vi "Timer Updated.vi"(8 "error in (no error)":errorcluster, 10 "Timer":timestamp format="%^<%H:%M:%S%3u>T", 11 "Module ID":i32=-1) -> (0 "error out":errorcluster)   [LabVIEW 2018, in "Timer Module.lvlib"]
doc: "Timer module broadcasts every time the timer increments its value.\n_____\nCreated using Delacor QMH Event Scripter 4.1.0.76."
uses:
  Timer Module.lvlib
  Timer Updated Argument--cluster.ctl
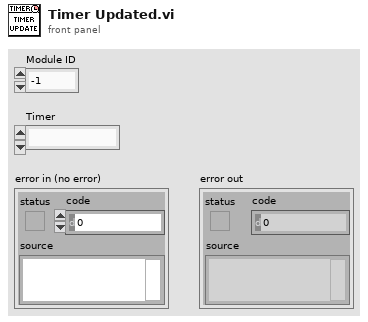
[diagram p1: front panel]
types:
  T1 = typedef "Timer Module.lvlib/Timer Updated Argument--cluster.ctl" = cluster{"Module ID":i32, "Timer":timestamp}
  T2 = typedef "Timer Module.lvlib/Broadcast Events--cluster.ctl" = cluster{"Module Did Init":refnum<user-event>, "Status Updated":refnum<user-event>, "Error Reported":refnum<user-event>, "Module Did Stop":refnum<user-event>, "Update Module Execution Status":refnum<user-event>, "Timer Updated":refnum<user-event>}
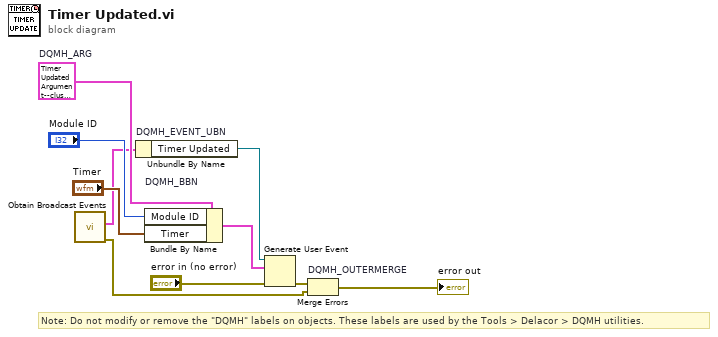
[diagram p0: block diagram]
diagram:
  w5 = T1 {"Module ID"=-1, "Timer"=timestamp(0 s since 1904-01-01)}  # DQMH_ARG
  # "Note: Do not modify or remove the \"DQMH\" labels on objects. These labels are used by the Tools > Delacor > DQMH utilities."
  n1 = call "Obtain Broadcast Events.vi"() -> ("error out"=w2:errorcluster, "Timer Module Broadcast Events"=w1:T2)  [unwired: 10 in]
  n2 = Unbundle By Name "DQMH_EVENT_UBN"(w1) -> ("Timer Updated"=w7:refnum<user-event>)
  n3 = Bundle By Name "DQMH_BBN"(cluster=w5, "Module ID"="Module ID", "Timer"="Timer") -> (w8:T1)
  n4 = Generate User Event(user event=w7, event data cluster=w8, error in="error in (no error)") -> (error out=w6:errorcluster)  [unwired: 1 in, 1 out]
  n5 = Merge Errors "DQMH_OUTERMERGE"(w6, w2) -> (→"error out":errorcluster)
